vi "ELVIS III v1.0 DO Build Bank Data.vi"(8 "error in (no error)":errorcluster, 9 "Wait Until Done?":bool, 10 "Channel Bitmask":bool[](array[boolean]), 11 "Bank Data":bool[][](array[boolean])) -> (0 "error out":errorcluster, 1 "Channel Selected?":bool, 3 "Bank Data":T1 caption="DO (N Samples) Configuration")   [LabVIEW 2021]
uses:
  <vilib>/myRIO/Common/Instrument Driver Framework/ELVIS III v1.0/DO Block/typedefs/ELVIS III DO Block Bank Data.ctl
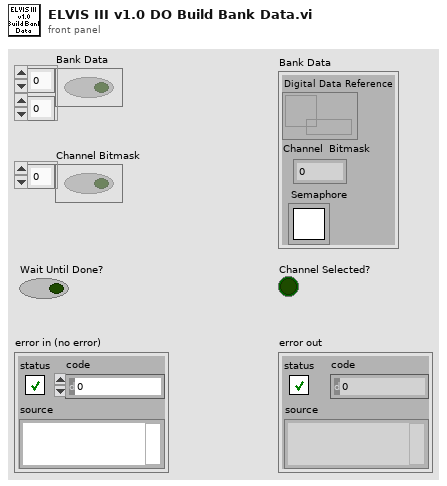
[diagram p1: front panel]
types:
  T1 = typedef "ELVIS III DO Block Bank Data.ctl" = cluster{"Digital Data Reference":refnum<data-value>, "Channel  Bitmask":fxp<+,20,20>, "Semaphore":T2}
  T2 = typedef "Semaphore RefNum" = refnum<k1>
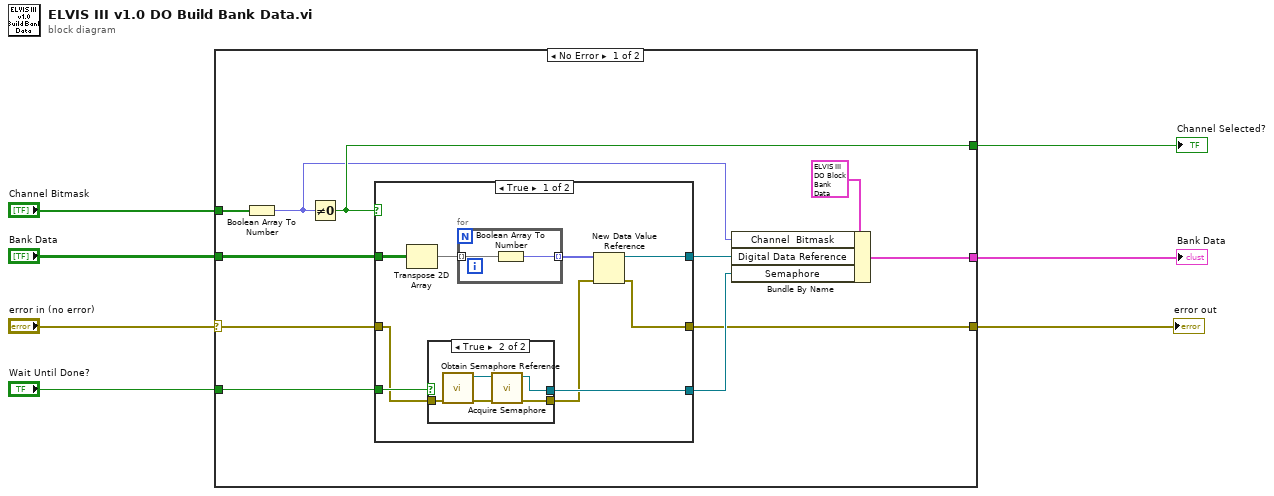
[diagram p0: block diagram]
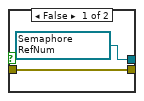
[diagram p2: hidden frame]
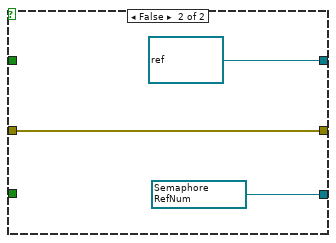
[diagram p3: hidden frame]
diagram:
  n1 = case shown="No Error" "error in (no error)" {
    selector: "error in (no error)" -> [w9 w40]
    tunnel: "Channel Bitmask" -> [w18 _]
    tunnel: [w17 _] -> w6
    tunnel: "Wait Until Done?" -> [w16 _]
    tunnel: "Bank Data" -> [w15 _]
    tunnel: [w10 _] -> w3
    tunnel: [w8 w40] -> w1
    frame No Error {
      n2 = Boolean Array To Number(Boolean array=w18) -> (number=w11:fxp<+,20,20>)
      n3 = Not Equal To 0?(x=w11) -> (x != 0?=w17:bool)
      n4 = case shown="True" w17 {
        tunnel: [w23 refnum<data-value> refnum ("data value reference")] -> w13
        tunnel: [w22 w37] -> w12
        tunnel: w16 -> [w27 _]
        tunnel: w15 -> [w25 _]
        tunnel: w9 -> [w20 w38]
        tunnel: [w21 w38] -> w8
        frame True {
          n5 = Transpose 2D Array(2D array=w25) -> (transposed array=w26:bool[][])
          n6 = case shown="True" w27 {
            tunnel: [w31 w32] -> w22
            tunnel: w20 -> [w30 w36]
            tunnel: [w30 w34] -> w19
            frame False {
              w31 = T2 refnum items=["semaphore"] ("semaphore out")
            }
            frame True {
              n7 = call <vilib>:"Obtain Semaphore Reference.vi"("error in (no error)"=w36) -> ("error out"=w35:errorcluster, "semaphore"=w33:T2)  [unwired: 4 in, 1 out]
              n8 = call <vilib>:"Acquire Semaphore.vi"("error in (no error)"=w35, "semaphore"=w33) -> ("error out"=w34:errorcluster, "semaphore out"=w32:T2)  [unwired: 3 in, 1 out]
            }
          }
          n9 = for {
            tunnel: w26 -> [w29] mode=indexing
            tunnel: [w28] -> w24 mode=indexing
            n10 = Boolean Array To Number(Boolean array=w29) -> (number=w28:fxp<+,20,20>)
          }
          n11 = New Data Value Reference(data value=w24, error in=w19) -> (data value reference=w23:refnum<data-value>, error out=w21:errorcluster)
        }
        frame False {
          w37 = T2 refnum items=["semaphore"] ("semaphore out")
        }
      }
      n12 = Bundle By Name(cluster=T1 {"Digital Data Reference"=refnum, "Channel  Bitmask"=0.0, "Semaphore"=refnum} ("DO (N Samples) Bank Configuration"), "Channel  Bitmask"=w11, "Digital Data Reference"=w13, "Semaphore"=w12) -> (w10:T1)
    }
    frame Error {
    }
  }
  "Bank Data" <- w3
  "Channel Selected?" <- w6
  "error out" <- w1
